vi "Configuration writer.vi"(0 "Path":T1, 1 "Width (px)":i32=240, 2 "error in (no error)":errorcluster, 3 "Precision (%)":dbl=1.0 min=1.0 max=100.0 step=1.0 format="%#_3g", 4 "Heigth (px)":i32=240, 5 "X offset":i32=693 step=1, 6 "X travel":dbl min=0.0 max=50.0 step=0.0001, 7 "Y offset":i32=406 step=1, 10 "Speed (µm/s)":i32=1000, 11 "Height  step \ndivider":i32=2, 12 "Y travel":dbl min=0.0 max=5.0 step=0.0001, 13 "Pixel size":dbl=12.19 step=0.01, 14 "Pixelclock":i32(slide)=24 min=5 max=40 step=1 scale=5.0..40.0, 15 "Framerate":dbl(slide)=10.002522802986672 min=0.47411700449083627 max=15.001275108384213 step=0.014032998230481021 scale=0.47411700449083627..15.001275108384213 scale format="%#.3g", 17 "Exposure":dbl(slide)=99.80425000000001 min=0.06241666666666667 max=99.80425000000001 step=0.06241666666666667 scale=0.06241666666666667..99.80425000000001 scale format="%#.3g") -> (19 "error out":errorcluster)   [LabVIEW 2016]
uses:
  <vilib>/Utility/config.llb/Config Data RefNum.ctl
  <vilib>/Utility/config.llb/Write Key (Double).vi
  <vilib>/Utility/config.llb/Write Key (I32).vi
  <vilib>/Utility/config.llb/NI_LVConfig.lvlib
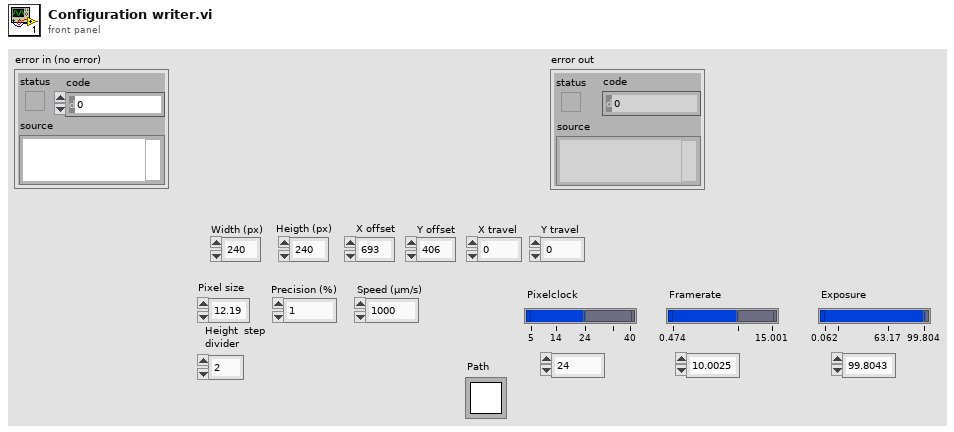
[diagram p1: front panel]
types:
  T1 = typedef "NI_LVConfig.lvlib/Config Data RefNum.ctl" = refnum<k1>
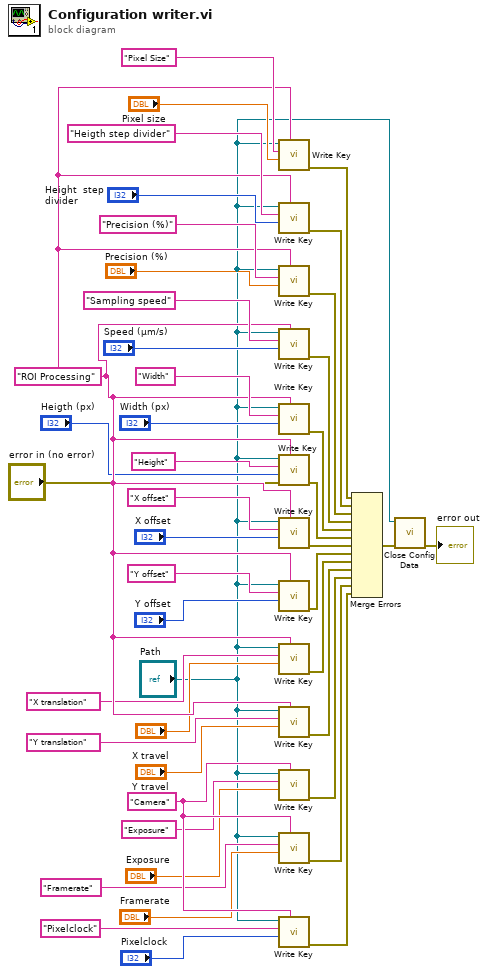
[diagram p0: block diagram]
diagram:
  w11 = "Camera" ("section")
  w28 = "ROI Processing" ("section")
  n1 = call-poly <vilib>:"Write Key.vi"("section"=w28, "value"="Pixel size", "key"="Pixel Size", "refnum"="Path") -> ("error out"=w37:errorcluster)  [unwired: 5 in, 2 out]
  n2 = call-poly <vilib>:"Write Key.vi"("section"=w28, "value"="Height  step \ndivider", "key"="Heigth step divider", "refnum"="Path") -> ("error out"=w36:errorcluster)  [unwired: 5 in, 2 out]
  n3 = call-poly <vilib>:"Write Key.vi"("section"=w28, "value"="Precision (%)", "key"="Precision (%)", "refnum"="Path") -> ("error out"=w35:errorcluster)  [unwired: 5 in, 2 out]
  n4 = call-poly <vilib>:"Write Key.vi"("section"=w28, "value"="Speed (µm/s)", "key"="Sampling speed", "refnum"="Path") -> ("error out"=w34:errorcluster)  [unwired: 5 in, 2 out]
  n5 = call-poly <vilib>:"Write Key.vi"("section"=w28, "value"="Width (px)", "key"="Width", "refnum"="Path") -> ("error out"=w33:errorcluster)  [unwired: 5 in, 2 out]
  n6 = call-poly <vilib>:"Write Key.vi"("section"=w28, "error in (no error)"="error in (no error)", "value"="Heigth (px)", "key"="Height", "refnum"="Path") -> ("error out"=w32:errorcluster)  [unwired: 4 in, 2 out]
  n7 = call-poly <vilib>:"Write Key.vi"("section"=w28, "value"="X offset", "key"="X offset", "refnum"="Path") -> ("error out"=w31:errorcluster)  [unwired: 5 in, 2 out]
  n8 = call-poly <vilib>:"Write Key.vi"("section"=w28, "value"="Y offset", "key"="Y offset", "refnum"="Path") -> ("error out"=w30:errorcluster)  [unwired: 5 in, 2 out]
  n9 = call-poly <vilib>:"Write Key.vi"("section"=w28, "value"="X travel", "key"="X translation", "refnum"="Path") -> ("error out"=w25:errorcluster)  [unwired: 5 in, 2 out]
  n10 = call-poly <vilib>:"Write Key.vi"("section"=w28, "value"="Y travel", "key"="Y translation", "refnum"="Path") -> ("error out"=w24:errorcluster)  [unwired: 5 in, 2 out]
  n11 = call-poly <vilib>:"Write Key.vi"("section"=w11, "value"="Exposure", "key"="Exposure", "refnum"="Path") -> ("error out"=w2:errorcluster)  [unwired: 5 in, 2 out]
  n12 = call-poly <vilib>:"Write Key.vi"("section"=w11, "value"="Framerate", "key"="Framerate", "refnum"="Path") -> ("error out"=w3:errorcluster)  [unwired: 5 in, 2 out]
  n13 = call-poly <vilib>:"Write Key.vi"("section"=w11, "value"="Pixelclock", "key"="Pixelclock", "refnum"="Path") -> ("error out"=w4:errorcluster)  [unwired: 5 in, 2 out]
  n14 = Merge Errors(w37, w36, w35, w34, w33, w32, w31, w30, w25, w24, w2, w3, w4) -> (w29:errorcluster)
  n15 = call <vilib>:"Close Config Data.vi"("error in (no error)"=w29, "refnum"="Path") -> ("error out"=→"error out":errorcluster)  [unwired: 8 in, 1 out]
